vi "SDGETPort.vi"(8 "error in (no error)":errorcluster, 10 "Expected response":string, 11 "UI Actor in":refnum<class "UI Actor.lvclass">) -> (0 "error out":errorcluster)   [LabVIEW 2020, in "UI Actor.lvlib" / "UI Actor.lvclass"]
doc: "Dependiendo del comando que se obtenga serial para saber el valor del puerto es traducido en leds que se muestran en Actor core con ayuda de eventos"
uses:
  UI Actor.lvclass
  UI Actor.lvclass/UI Actor.ctl
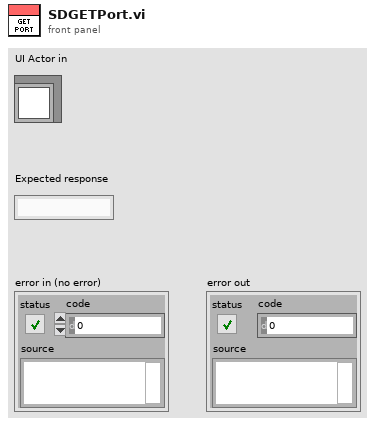
[diagram p1: front panel]
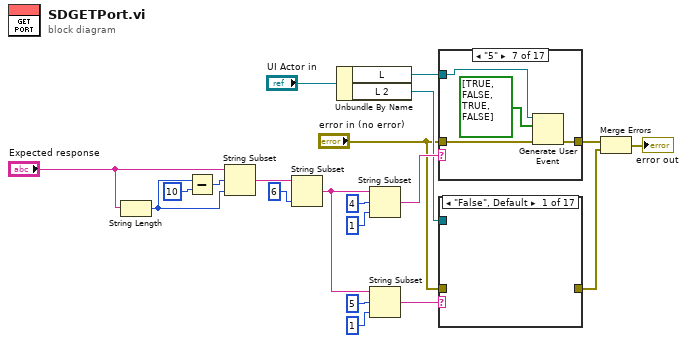
[diagram p0: block diagram]
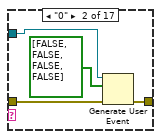
[diagram p2: hidden frame]
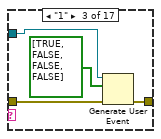
[diagram p3: hidden frame]
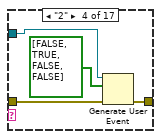
[diagram p4: hidden frame]
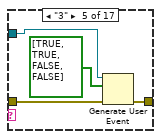
[diagram p5: hidden frame]
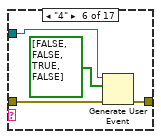
[diagram p6: hidden frame]
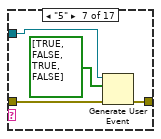
[diagram p7: hidden frame]
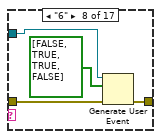
[diagram p8: hidden frame]
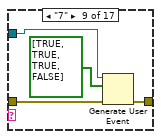
[diagram p9: hidden frame]
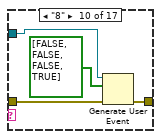
[diagram p10: hidden frame]
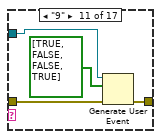
[diagram p11: hidden frame]
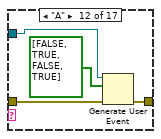
[diagram p12: hidden frame]
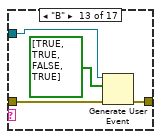
[diagram p13: hidden frame]
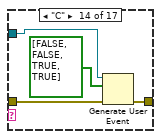
[diagram p14: hidden frame]
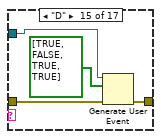
[diagram p15: hidden frame]
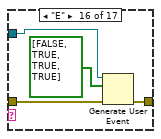
[diagram p16: hidden frame]
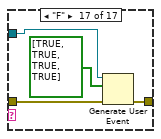
[diagram p17: hidden frame]
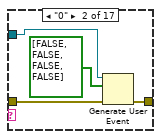
[diagram p19: hidden frame]
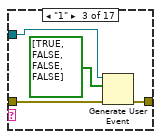
[diagram p20: hidden frame]
diagram:
  n1 = String Length(string="Expected response") -> (length=w15:i32)
  n2 = Subtract(x=w15, y=10) -> (x-y=w16:i32)
  n3 = String Subset(string="Expected response", offset (0)=w16, length (rest)=w15) -> (substring=w14:string)
  n4 = String Subset(string=w14, length (rest)=6 ("length (rest)")) -> (substring=w7:string)  [unwired: 1 in]
  n5 = Unbundle By Name("UI Actor in") -> ("L"=w19:refnum<user-event>, "L 2"=w6:refnum<user-event>)
  n6 = String Subset(string=w7, offset (0)=4, length (rest)=1 ("length (rest)")) -> (substring=w10:string)
  n7 = String Subset(string=w7, offset (0)=5, length (rest)=1 ("length (rest)")) -> (substring=w2:string)
  n8 = case shown="\"5\"" w10 {
    tunnel: w19 -> [_ w24 w28 w32 w36 w40 w44 w48 w52 w56 w60 w64 w68 w72 w76 w80 w84]
    tunnel: "error in (no error)" -> [_ w22 w26 w30 w34 w38 w42 w46 w50 w54 w58 w62 w66 w70 w74 w78 w82]
    tunnel: [_ w21 w25 w29 w33 w37 w41 w45 w49 w53 w57 w61 w65 w69 w73 w77 w81] -> w20
    frame "False", Default {
    }
    frame "0" {
      n9 = Generate User Event(user event=w24, event data cluster=bool[] [FALSE, FALSE, FALSE, FALSE] ("event data"), error in=w22) -> (error out=w21:errorcluster)  [unwired: 1 in, 1 out]
    }
    frame "1" {
      n10 = Generate User Event(user event=w28, event data cluster=bool[] [TRUE, FALSE, FALSE, FALSE] ("event data"), error in=w26) -> (error out=w25:errorcluster)  [unwired: 1 in, 1 out]
    }
    frame "2" {
      n11 = Generate User Event(user event=w32, event data cluster=bool[] [FALSE, TRUE, FALSE, FALSE] ("event data"), error in=w30) -> (error out=w29:errorcluster)  [unwired: 1 in, 1 out]
    }
    frame "3" {
      n12 = Generate User Event(user event=w36, event data cluster=bool[] [TRUE, TRUE, FALSE, FALSE] ("event data"), error in=w34) -> (error out=w33:errorcluster)  [unwired: 1 in, 1 out]
    }
    frame "4" {
      n13 = Generate User Event(user event=w40, event data cluster=bool[] [FALSE, FALSE, TRUE, FALSE] ("event data"), error in=w38) -> (error out=w37:errorcluster)  [unwired: 1 in, 1 out]
    }
    frame "5" {
      n14 = Generate User Event(user event=w44, event data cluster=bool[] [TRUE, FALSE, TRUE, FALSE] ("event data"), error in=w42) -> (error out=w41:errorcluster)  [unwired: 1 in, 1 out]
    }
    frame "6" {
      n15 = Generate User Event(user event=w48, event data cluster=bool[] [FALSE, TRUE, TRUE, FALSE] ("event data"), error in=w46) -> (error out=w45:errorcluster)  [unwired: 1 in, 1 out]
    }
    frame "7" {
      n16 = Generate User Event(user event=w52, event data cluster=bool[] [TRUE, TRUE, TRUE, FALSE] ("event data"), error in=w50) -> (error out=w49:errorcluster)  [unwired: 1 in, 1 out]
    }
    frame "8" {
      n17 = Generate User Event(user event=w56, event data cluster=bool[] [FALSE, FALSE, FALSE, TRUE] ("event data"), error in=w54) -> (error out=w53:errorcluster)  [unwired: 1 in, 1 out]
    }
    frame "9" {
      n18 = Generate User Event(user event=w60, event data cluster=bool[] [TRUE, FALSE, FALSE, TRUE] ("event data"), error in=w58) -> (error out=w57:errorcluster)  [unwired: 1 in, 1 out]
    }
    frame "A" {
      n19 = Generate User Event(user event=w64, event data cluster=bool[] [FALSE, TRUE, FALSE, TRUE] ("event data"), error in=w62) -> (error out=w61:errorcluster)  [unwired: 1 in, 1 out]
    }
    frame "B" {
      n20 = Generate User Event(user event=w68, event data cluster=bool[] [TRUE, TRUE, FALSE, TRUE] ("event data"), error in=w66) -> (error out=w65:errorcluster)  [unwired: 1 in, 1 out]
    }
    frame "C" {
      n21 = Generate User Event(user event=w72, event data cluster=bool[] [FALSE, FALSE, TRUE, TRUE] ("event data"), error in=w70) -> (error out=w69:errorcluster)  [unwired: 1 in, 1 out]
    }
    frame "D" {
      n22 = Generate User Event(user event=w76, event data cluster=bool[] [TRUE, FALSE, TRUE, TRUE] ("event data"), error in=w74) -> (error out=w73:errorcluster)  [unwired: 1 in, 1 out]
    }
    frame "E" {
      n23 = Generate User Event(user event=w80, event data cluster=bool[] [FALSE, TRUE, TRUE, TRUE] ("event data"), error in=w78) -> (error out=w77:errorcluster)  [unwired: 1 in, 1 out]
    }
    frame "F" {
      n24 = Generate User Event(user event=w84, event data cluster=bool[] [TRUE, TRUE, TRUE, TRUE] ("event data"), error in=w82) -> (error out=w81:errorcluster)  [unwired: 1 in, 1 out]
    }
  }
  n25 = case shown="\"False\", Default" w2 {
    tunnel: w6 -> [_ w88 w92 w96 w100 w104 w108 w112 w116 w120 w124 w128 w132 w136 w140 w144 w148]
    tunnel: "error in (no error)" -> [_ w86 w90 w94 w98 w102 w106 w110 w114 w118 w122 w126 w130 w134 w138 w142 w146]
    tunnel: [_ w85 w89 w93 w97 w101 w105 w109 w113 w117 w121 w125 w129 w133 w137 w141 w145] -> w3
    frame "False", Default {
    }
    frame "0" {
      n26 = Generate User Event(user event=w88, event data cluster=bool[] [FALSE, FALSE, FALSE, FALSE] ("event data"), error in=w86) -> (error out=w85:errorcluster)  [unwired: 1 in, 1 out]
    }
    frame "1" {
      n27 = Generate User Event(user event=w92, event data cluster=bool[] [TRUE, FALSE, FALSE, FALSE] ("event data"), error in=w90) -> (error out=w89:errorcluster)  [unwired: 1 in, 1 out]
    }
    frame "2" {
      n28 = Generate User Event(user event=w96, event data cluster=bool[] [FALSE, TRUE, FALSE, FALSE] ("event data"), error in=w94) -> (error out=w93:errorcluster)  [unwired: 1 in, 1 out]
    }
    frame "3" {
      n29 = Generate User Event(user event=w100, event data cluster=bool[] [TRUE, TRUE, FALSE, FALSE] ("event data"), error in=w98) -> (error out=w97:errorcluster)  [unwired: 1 in, 1 out]
    }
    frame "4" {
      n30 = Generate User Event(user event=w104, event data cluster=bool[] [FALSE, FALSE, TRUE, FALSE] ("event data"), error in=w102) -> (error out=w101:errorcluster)  [unwired: 1 in, 1 out]
    }
    frame "5" {
      n31 = Generate User Event(user event=w108, event data cluster=bool[] [TRUE, FALSE, TRUE, FALSE] ("event data"), error in=w106) -> (error out=w105:errorcluster)  [unwired: 1 in, 1 out]
    }
    frame "6" {
      n32 = Generate User Event(user event=w112, event data cluster=bool[] [FALSE, TRUE, TRUE, FALSE] ("event data"), error in=w110) -> (error out=w109:errorcluster)  [unwired: 1 in, 1 out]
    }
    frame "7" {
      n33 = Generate User Event(user event=w116, event data cluster=bool[] [TRUE, TRUE, TRUE, FALSE] ("event data"), error in=w114) -> (error out=w113:errorcluster)  [unwired: 1 in, 1 out]
    }
    frame "8" {
      n34 = Generate User Event(user event=w120, event data cluster=bool[] [FALSE, FALSE, FALSE, TRUE] ("event data"), error in=w118) -> (error out=w117:errorcluster)  [unwired: 1 in, 1 out]
    }
    frame "9" {
      n35 = Generate User Event(user event=w124, event data cluster=bool[] [TRUE, FALSE, FALSE, TRUE] ("event data"), error in=w122) -> (error out=w121:errorcluster)  [unwired: 1 in, 1 out]
    }
    frame "A" {
      n36 = Generate User Event(user event=w128, event data cluster=bool[] [FALSE, TRUE, FALSE, TRUE] ("event data"), error in=w126) -> (error out=w125:errorcluster)  [unwired: 1 in, 1 out]
    }
    frame "B" {
      n37 = Generate User Event(user event=w132, event data cluster=bool[] [TRUE, TRUE, FALSE, TRUE] ("event data"), error in=w130) -> (error out=w129:errorcluster)  [unwired: 1 in, 1 out]
    }
    frame "C" {
      n38 = Generate User Event(user event=w136, event data cluster=bool[] [FALSE, FALSE, TRUE, TRUE] ("event data"), error in=w134) -> (error out=w133:errorcluster)  [unwired: 1 in, 1 out]
    }
    frame "D" {
      n39 = Generate User Event(user event=w140, event data cluster=bool[] [TRUE, FALSE, TRUE, TRUE] ("event data"), error in=w138) -> (error out=w137:errorcluster)  [unwired: 1 in, 1 out]
    }
    frame "E" {
      n40 = Generate User Event(user event=w144, event data cluster=bool[] [FALSE, TRUE, TRUE, TRUE] ("event data"), error in=w142) -> (error out=w141:errorcluster)  [unwired: 1 in, 1 out]
    }
    frame "F" {
      n41 = Generate User Event(user event=w148, event data cluster=bool[] [TRUE, TRUE, TRUE, TRUE] ("event data"), error in=w146) -> (error out=w145:errorcluster)  [unwired: 1 in, 1 out]
    }
  }
  n42 = Merge Errors(w20, w3) -> (→"error out":errorcluster)
